vi "Main-loop-with-queues.vi"() -> ()   [LabVIEW 2016]
uses:
  <vilib>/Platform/TimedLoop/XDataNode/XDataNode.xnode
  <vilib>/Platform/TimedLoop/XDataNode/nitl_modes.ctl
  <vilib>/Platform/TimedLoop/XDataNode/XDNodeRunTimeDep.lvlib
  <vilib>/Platform/TimedLoop/XDataNode/wakeup.ctl
  <vilib>/Platform/TimedLoop/XDataNode/timing_clust.ctl
  Plant_info.ctl
  Sched_state.ctl
panel:
  out "Numeric":i32
  out "Region Plant 1":i32
  out "Region Plant 2":i32
  in  "stop":bool
  out "error out":errorcluster
  in  "error in (no error)":errorcluster
  in  "stop main":bool
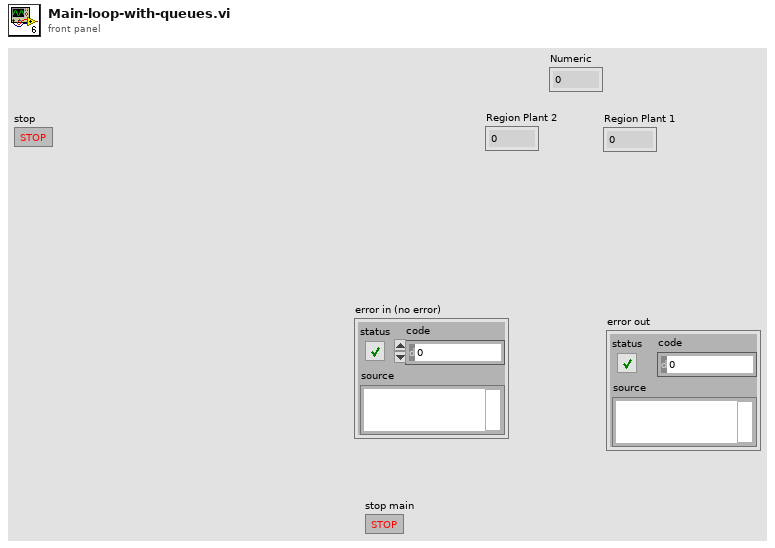
[diagram p1: front panel]
types:
  T1 = typedef "Sched_state.ctl" = cluster{"Plant 1":T2, "Plant 2":T2}
  T2 = typedef "Plant_info.ctl" = cluster{"Clk":dbl, "Region":dbl, "Input":dbl}
  T3 = typedef "Sched_queues.ctl" = cluster{"last region":refnum<queue>, "last state":refnum<queue>}
  T4 = typedef "XDNodeRunTimeDep.lvlib/timing_clust.ctl" = cluster{"Expected End [f-1]":u64, "Actual End [f-1]":u64, "Finished Late? [f-1]":bool, "Expected End [i-1]":u64, "Actual End [i-1]":u64, "Finished Late? [i-1]":bool, "Expected Start [i]":u64, "Actual Start [i]":u64, "Expected Start [f]":u64, "Actual Start [f]":u64, "Source Name":string, "Structure Name":string, "Period":i64, "Deadline":i64, "Offset":i64, "Start":i64, "Priority":i32, "Timeout":i32, "Mode":T5, "Wakeup Reason":T6, "Error":errorcluster, "Source Type":string, "Secondary Source Type":string, "Global End Time":u64, "Global Start Time":u64, "Frame Duration":u64, "Iteration Duration":u64, "Assigned CPU":i32, "I/O Scan Engine Mode":u32}
  T5 = typedef "XDNodeRunTimeDep.lvlib/nitl_modes.ctl" = enum32{"No Change", "Process missed periods, maintain original phase", "Discard missed periods, maintain original phase", "Process missed periods, ignore original phase", "Discard missed periods, ignore original phase"}
  T6 = typedef "XDNodeRunTimeDep.lvlib/wakeup.ctl" = enum32{"Normal", "Aborted", "Asynchronous wakeup", "Timing source error", "Timed loop error", "Timeout"}
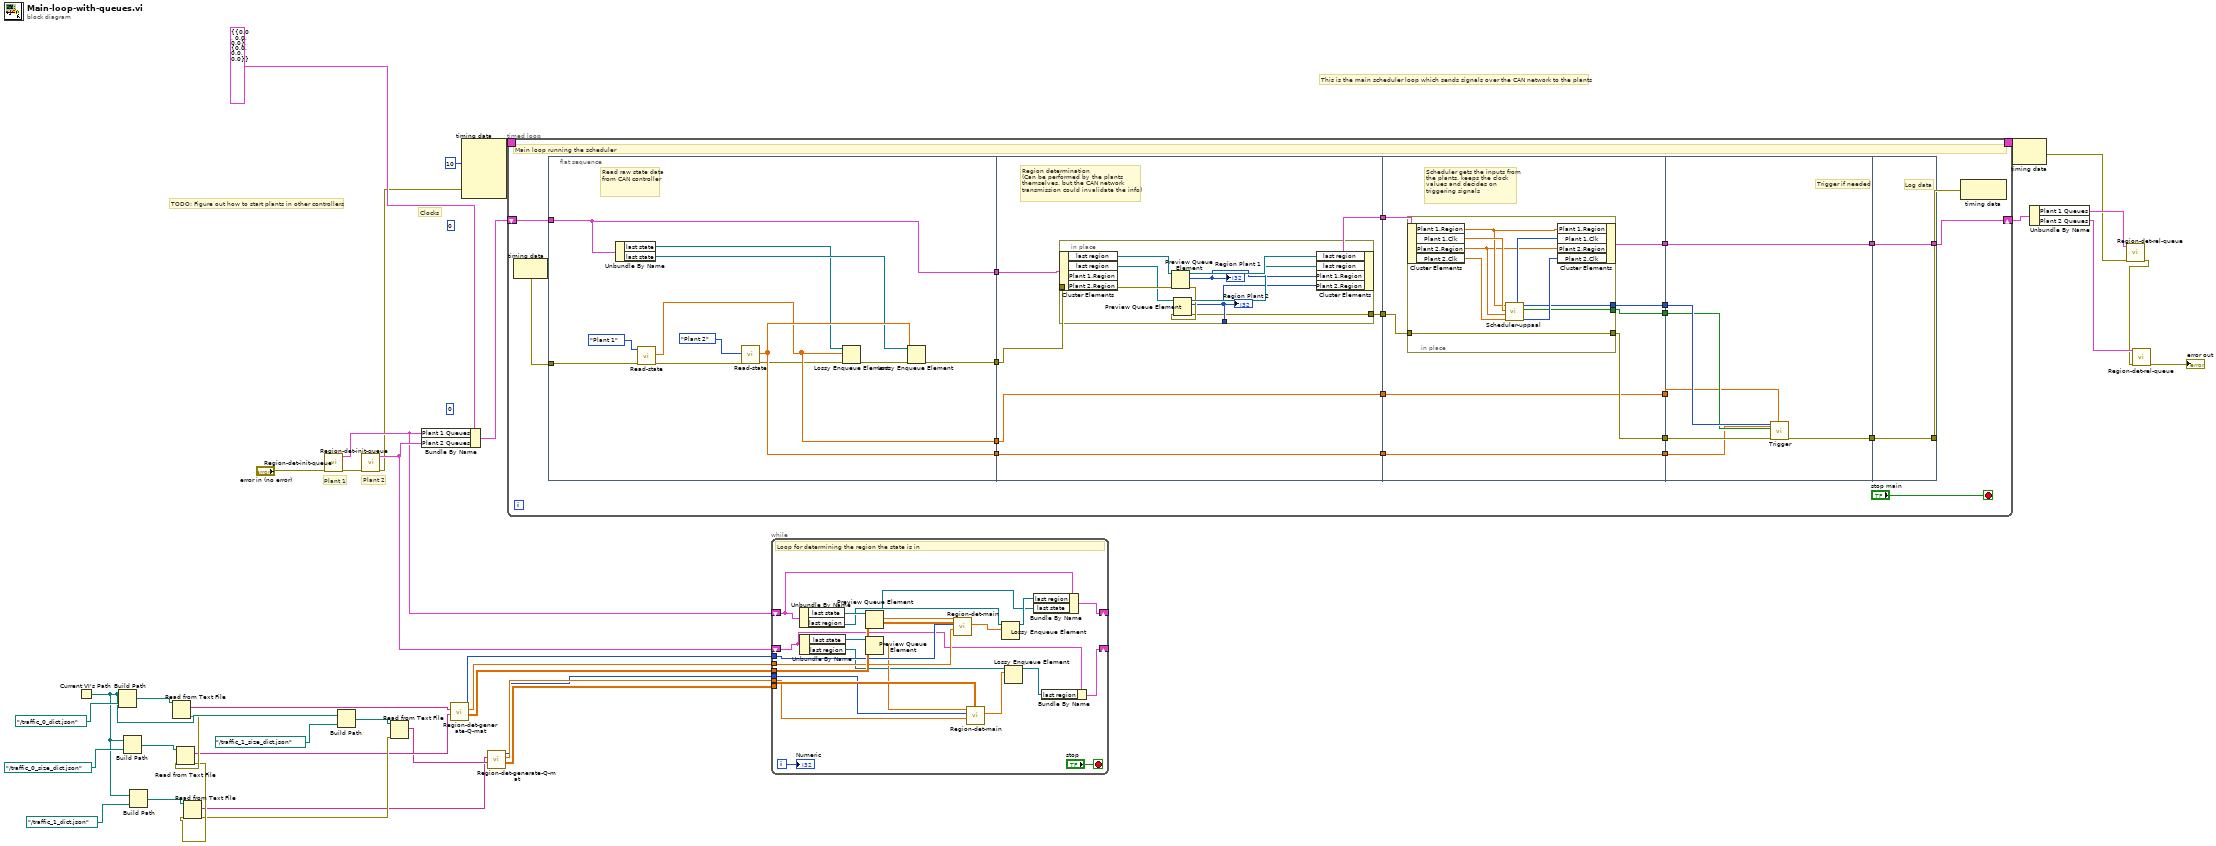
[diagram p0: block diagram]
diagram:
  (unwired) 0
  (unwired) 0
  # "Plant 1"
  # "Plant 2"
  # "Clocks"
  # "TODO: Figure out how to start plants in other controllers"
  # "This is the main scheduler loop which sends signals over the CAN network to the plants"
  n1 = Current VI's Path() -> (path=w21:path)
  n2 = Build Path(base path=w21, name or relative path=path "../traffic_0_dict.json") -> (appended path=w29:path)
  n3 = Build Path(base path=w21, name or relative path=path "../traffic_0_size_dict.json") -> (appended path=w26:path)
  n4 = Build Path(base path=w21, name or relative path=path "../traffic_1_dict.json") -> (appended path=w25:path)
  n5 = Read from Text File(file (use dialog)=w29) -> (text=w17:string, error out=w20:errorcluster)  [unwired: 3 in, 2 out]
  n6 = Read from Text File(file (use dialog)=w26, error in=w20) -> (text=w16:string, error out=w19:errorcluster)  [unwired: 2 in, 2 out]
  n7 = Read from Text File(file (use dialog)=w25, error in=w19) -> (text=w14:string, error out=w18:errorcluster)  [unwired: 2 in, 2 out]
  n8 = call "Region-det-init-queue.vi"("error in (no error)"="error in (no error)") -> ("error out"=w33:errorcluster, "Queues"=w30:T3)  [unwired: 9 in]
  n9 = Build Path(base path=w21, name or relative path=path "../traffic_1_size_dict.json") -> (appended path=w22:path)
  n10 = call "Region-det-init-queue.vi"("error in (no error)"=w33) -> ("error out"=w1:errorcluster, "Queues"=w31:T3)  [unwired: 9 in]
  n11 = Read from Text File(file (use dialog)=w22, error in=w18) -> (text=w15:string)  [unwired: 2 in, 3 out]
  n12 = Bundle By Name(cluster=T1 {"Plant 1"={"Clk"=0.0, "Region"=0.0, "Input"=0.0}, "Plant 2"={"Clk"=0.0, "Region"=0.0, "Input"=0.0}} ("Scheduler State"), "Plant 1 Queues"=w30, "Plant 2 Queues"=w31) -> (w32:T1)
  n13 = call "Region-det-generate-Q-mat.vi"("Q region size JSON string"=w16, "Q matrix JSON string"=w17) -> ("Q Matrices"=w12:dbl[][][][], "Index array"=w13:dbl[], "Regions"=w9:i32[])  [unwired: 6 in, 1 out]
  n14 = node-c288(i64 10 ("Period"), w1) -> (w38:T4)  [unwired: 3 in]
  n15 = call "Region-det-generate-Q-mat.vi"("Q region size JSON string"=w15, "Q matrix JSON string"=w14) -> ("Q Matrices"=w10:dbl[][][][], "Index array"=w11:dbl[], "Regions"=w8:i32[])  [unwired: 6 in, 1 out]
  n16 = timed-loop {
    timing: w38 -> [_]
    timing-out: [_] -> w37
    shift-right: [w39] -> w7
    shift-left: w32 -> [w56]
    stop <- "stop main" stop-if-true
    # "Main loop running the scheduler"
    n17 = node-c288() -> (w59:errorcluster)  [unwired: 1 in]
    n18 = flat-sequence {
      tunnel: w59 -> [w62]
      tunnel: w56 -> [w63]
      tunnel: [w71] -> w55
      tunnel: [w70] -> w49
      tunnel: [w65] -> w48
      tunnel: [w63] -> w40
      tunnel: w55 -> [w77]
      tunnel: [w76] -> w54
      tunnel: [w75] -> w51
      tunnel: w49 -> [w73]
      tunnel: w48 -> [w74]
      tunnel: [w74] -> w47
      tunnel: [w73] -> w44
      tunnel: w40 -> [w72]
      tunnel: w54 -> [w94]
      tunnel: [w93] -> w53
      tunnel: [w92] -> w52
      tunnel: w51 -> [w91]
      tunnel: [w90] -> w50
      tunnel: w47 -> [w89]
      tunnel: [w89] -> w46
      tunnel: [w88] -> w45
      tunnel: w44 -> [w88]
      tunnel: [w87] -> w41
      tunnel: [w110] -> w58
      tunnel: w53 -> [w109]
      tunnel: w52 -> [w108]
      tunnel: w50 -> [w107]
      tunnel: w46 -> [w106]
      tunnel: w45 -> [w105]
      tunnel: [w104] -> w42
      tunnel: w41 -> [w104]
      tunnel: [w112] -> w43
      tunnel: w58 -> [w112]
      tunnel: [w111] -> w39
      tunnel: w42 -> [w111]
      frame #0 {
        # "Read raw state data from CAN controller"
        n19 = Unbundle By Name(w63) -> ("last state"=w64:refnum<queue>, "last state"=w69:refnum<queue>)
        n20 = call "Read-state.vi"("error in (no error)"=w62, "Plant"=enum16{"Plant 1", "Plant 2"}."Plant 1") -> ("error out"=w61:errorcluster, "state"=w65:dbl[])  [unwired: 8 in]
        n21 = call "Read-state.vi"("error in (no error)"=w61, "Plant"=enum16{"Plant 1", "Plant 2"}."Plant 2") -> ("error out"=w60:errorcluster, "state"=w70:dbl[])  [unwired: 8 in]
        n22 = Lossy Enqueue Element(queue=w64, element=w65, error in (no error)=w60) -> (error out=w66:errorcluster)  [unwired: 3 out]
        n23 = Lossy Enqueue Element(queue=w69, element=w70, error in (no error)=w66) -> (error out=w71:errorcluster)  [unwired: 3 out]
      }
      frame #1 {
        # "Region determination \n(Can be performed by the plants\nthemselves, but the CAN network \ntransmission could invalidate the info)"
        n24 = in-place {
          in-place-border: w77 -> [w84]
          in-place-border: [w81] -> _
          in-place-border: [w80] -> w75
          n25 = in-place-cluster #1(w72) -> ("last region"=w79:refnum<queue>, "last region"=w78:refnum<queue>)  [unwired: 2 out]
          n26 = Preview Queue Element(queue=w79, error in (no error)=w84) -> (queue out=w86:refnum<queue>, element=w82:i32, error out=w83:errorcluster)  [unwired: 1 in, 1 out]
          "Region Plant 1" <- w82
          n27 = Preview Queue Element(queue=w78, error in (no error)=w83) -> (queue out=w85:refnum<queue>, element=w81:i32, error out=w80:errorcluster)  [unwired: 1 in, 1 out]
          "Region Plant 2" <- w81
          n28 = in-place-cluster #1("last region"=w86, "last region"=w85, "Plant 1.Region"=w82, "Plant 2.Region"=w81) -> (w76:T1)
        }
      }
      frame #2 {
        # "Scheduler gets the inputs from the plants, keeps the clock values and decides on triggering signals"
        n29 = in-place {
          in-place-border: [w101] -> w93
          in-place-border: [w100] -> w92
          in-place-border: [w99] -> w90
          in-place-border: w91 -> [w99]
          n30 = in-place-cluster #2(w94) -> ("Plant 1.Region"=w96:dbl, "Plant 1.Clk"=w98:dbl, "Plant 2.Region"=w95:dbl, "Plant 2.Clk"=w97:dbl)
          n31 = call "Scheduler-uppaal.vi"("Clock, plant 2"=w97, "Region, plant 2"=w95, "Clock, plant 1"=w98, "Region, plant 1"=w96) -> ("Clock 2"=w102:i32, "Clock 1"=w103:i32, "Trigger?"=w100:bool, "Plant to trigg"=w101:enum16{"Plant 1", "Plant 2"})  [unwired: 4 in]
          n32 = in-place-cluster #2("Plant 1.Region"=w96, "Plant 1.Clk"=w103, "Plant 2.Region"=w95, "Plant 2.Clk"=w102) -> (w87:T1)
        }
      }
      frame #3 {
        # "Trigger if needed"
        n33 = call "Trigger.vi"(5:w105, 7:w106, "error in (no error)"=w107, "State, Plant 1"=w108, "Plant to trigg"=w109) -> ("error out"=w110:errorcluster)  [unwired: 5 in, 1 out]
      }
      frame #4 {
        # "Log data"
      }
    }
    n34 = node-c288(w43) -> ()  [unwired: 1 out]
  }
  n35 = while {
    tunnel: w13 -> [w135]
    tunnel: w12 -> [w138]
    tunnel: w11 -> [w131]
    tunnel: w10 -> [w134]
    tunnel: w9 -> [w136]
    tunnel: w8 -> [w132]
    shift-right: [w122] -> _
    shift-left: w30 -> [w123]
    shift-right: [w124] -> _
    shift-left: w31 -> [w125]
    i -> [w119]
    stop <- "stop" stop-if-true
    # "Loop for determining the region the state is in"
    n36 = Unbundle By Name(w123) -> ("last state"=w140:refnum<queue>, "last region"=w130:refnum<queue>)
    n37 = Unbundle By Name(w125) -> ("last state"=w139:refnum<queue>, "last region"=w129:refnum<queue>)
    n38 = Preview Queue Element(queue=w140) -> (queue out=w118:refnum<queue>, element=w137:dbl[])  [unwired: 2 in, 2 out]
    n39 = Preview Queue Element(queue=w139) -> (element=w133:dbl[])  [unwired: 2 in, 3 out]
    n40 = call "Region-det-main.vi"(7:w138, "Index Array"=w135, "Regions"=w136, "State"=w137) -> ("Region"=w127:dbl)  [unwired: 7 in]
    n41 = call "Region-det-main.vi"(7:w134, "Index Array"=w131, "Regions"=w132, "State"=w133) -> ("Region"=w128:dbl)  [unwired: 7 in]
    n42 = Lossy Enqueue Element(queue=w130, element=w127) -> (queue out=w121:refnum<queue>)  [unwired: 1 in, 3 out]
    n43 = Lossy Enqueue Element(queue=w129, element=w128) -> (queue out=w126:refnum<queue>)  [unwired: 1 in, 3 out]
    n44 = Bundle By Name(cluster=w123, "last region"=w121, "last state"=w118) -> (w122:T3)
    n45 = Bundle By Name(cluster=w125, "last region"=w126) -> (w124:T3)
    "Numeric" <- w119
  }
  n46 = node-c288(w37) -> (w3:errorcluster)
  n47 = Unbundle By Name(w7) -> ("Plant 1 Queues"=w6:T3, "Plant 2 Queues"=w5:T3)
  n48 = call "Region-det-rel-queue.vi"("error in (no error)"=w3, "Queues"=w6) -> ("error out"=w4:errorcluster)  [unwired: 9 in]
  n49 = call "Region-det-rel-queue.vi"("error in (no error)"=w4, "Queues"=w5) -> ("error out"=→"error out":errorcluster)  [unwired: 9 in]
